vi "Try2.vi"() -> ()   [LabVIEW 2021]
uses:
  Explore/ROS_Subs/ROSCtrl.ctl
panel:
  out "Cmd Line":string
  out "left over fixed":string
  out "Console":string
  in  "Next":bool
  in  "Book":enum32{"Welcome", "lightshow"}(tab)
  in  "Python version":string="3.7"
  in  "Raspberry Pi":T1={"IP Address"="192.168.86.144", "Username"="ubuntu", "password"="iRobot"}
  in  "Update":bool
  in  "LED Colors":u32[](array[colorbox])=[16711680, 327424, 393471, 15699456, 14811391, 64255]
  out "lightshow":string
  # "Welcome to ROS2 for Create3\n\nto get started, enter your IP, hit run,\nand click on Next"
  # "Pick your colors and hit update"
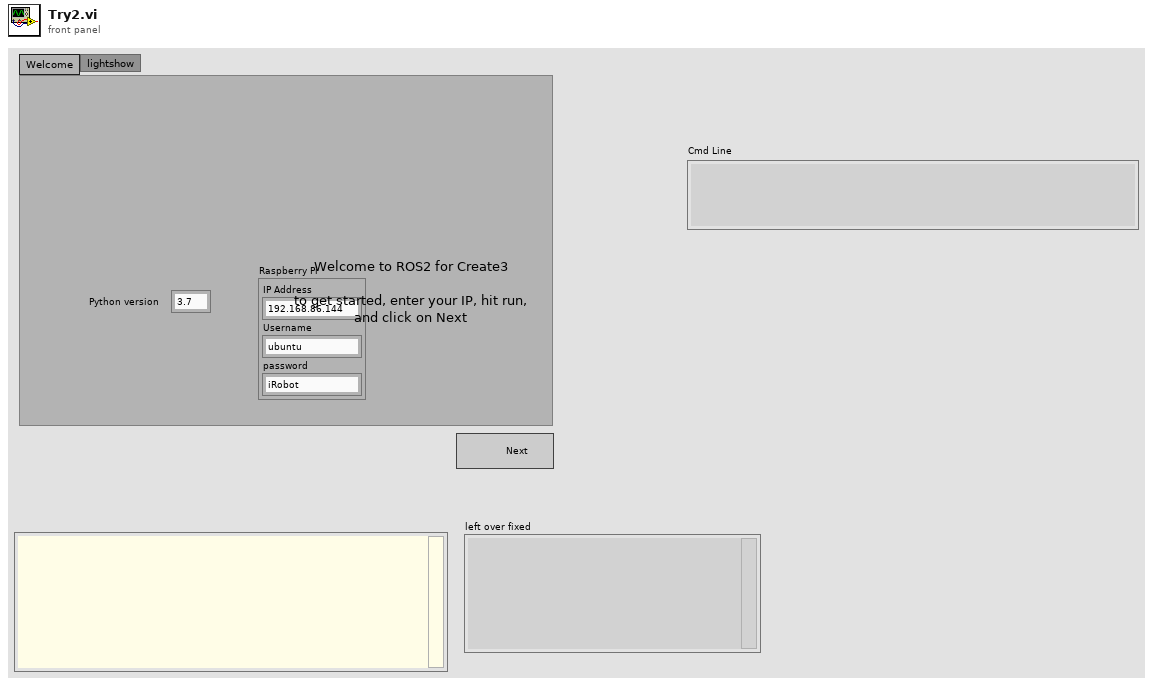
[diagram p1: front panel]
types:
  T1 = cluster{"IP Address":string, "Username":string, "password":string}
  T2 = typedef "ROSCtrl.ctl" = cluster{"Node Name":string, "Topic Name":string, "Message Type":string, "Message":string, "Pub_Time":string}
  T3 = cluster{"override_system":bool, "leds":cluster{"red":u8, "green":u8, "blue":u8}[]}
  T4 = typedef "PythonCtrl.ctl" = cluster{"session":refnum<k35>, "PyPath":path, "Processor":T5, "Port":string, "version":string}
  T5 = typedef "Processors.ctl" = enum16{"SPIKE", "Pi", "Pi_ssh", "OpenMV", "Dunio"}
  T6 = enum8{"Enabled", "Disabled", "Disabled and Grayed Out"}
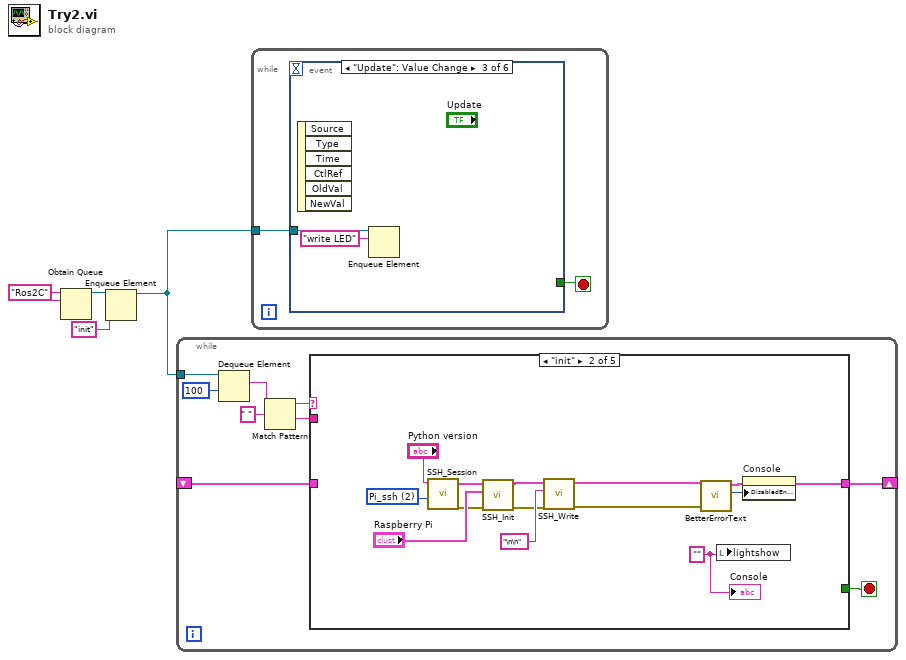
[diagram p0: block diagram]
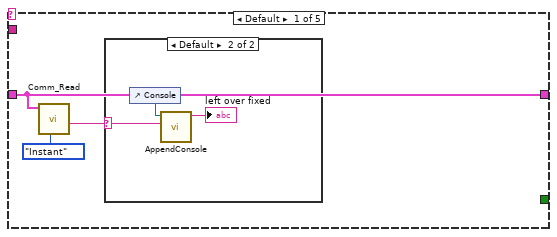
[diagram p2: hidden frame]
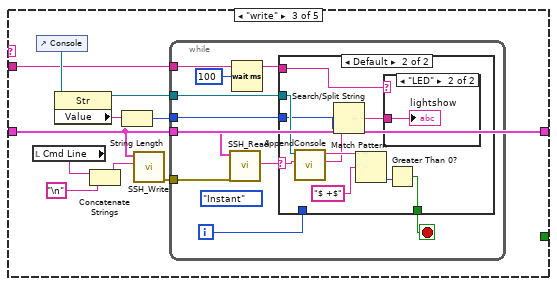
[diagram p4: hidden frame]
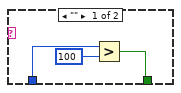
[diagram p5: hidden frame]
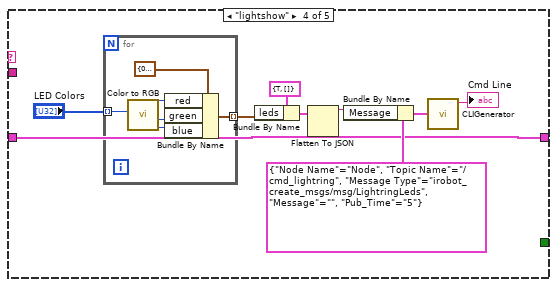
[diagram p7: hidden frame]
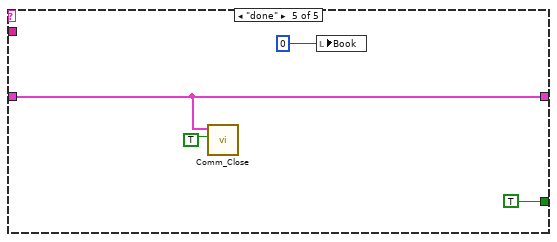
[diagram p8: hidden frame]
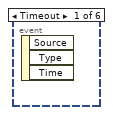
[diagram p9: hidden frame]
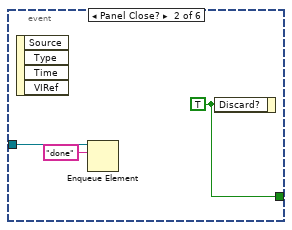
[diagram p10: hidden frame]
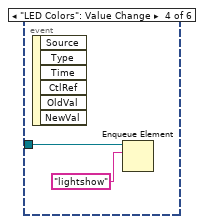
[diagram p11: hidden frame]
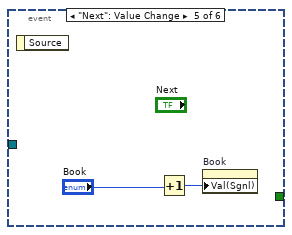
[diagram p12: hidden frame]
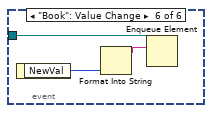
[diagram p13: hidden frame]
diagram:
  w4 = "Ros2C" ("name (unnamed)")
  n1 = Obtain Queue(name (unnamed)=w4, element data type=w4) -> (queue out=w3:refnum<queue>)  [unwired: 3 in, 2 out]
  n2 = Enqueue Element(queue=w3, element="init") -> (queue out=w2:refnum<queue>)  [unwired: 2 in, 2 out]
  n3 = while {
    tunnel: w2 -> [w12]
    shift-right: [w11] -> _
    shift-left: _ -> [w10]
    stop <- w13 stop-if-true
    n4 = Dequeue Element(queue=w12, timeout in ms (-1)=100) -> (element=w8:string)  [unwired: 1 in, 3 out]
    n5 = Match Pattern(string=w8, regular expression=" ") -> (before substring=w6:string, after substring=w5:string)  [unwired: 1 in, 2 out]
    n6 = case shown="\"init\"" w6 {
      tunnel: [_ _ _ _ TRUE ("Discard?")] -> w13
      tunnel: [w15 w31 w35 w65 w81] -> w11
      tunnel: w10 -> [w15 _ w35 w65 w81]
      tunnel: w5 -> [_ _ w36 _ _]
      frame Default {
        n7 = call "Comm_Read.vi"("Task"=enum16{"Instant", "All"}."Instant", "Python"=w15) -> ("Text read"=w14:string)  [unwired: 8 in, 1 out]
        n8 = case shown="Default" w14 {
          selector: w14 -> [_ w19]
          frame "" {
          }
          frame Default {
            n9 = control-ref of="Console"() -> (w18:refnum<vi>)
            n10 = call "AppendConsole.vi"("String"=w19, "String in"=w18) -> ("left over fixed"=→"left over fixed":string)  [unwired: 7 in, 2 out]
          }
        }
      }
      frame "init" {
        w20 = "" ("function name")
        w29 = u16 2 items=["SPIKE", "Pi", "Pi_ssh", "OpenMV", "duino"] ("Processor")
        n11 = call "SSH_Session.vi"("Processor"=w29, "Python version"="Python version") -> ("error out"=w26:errorcluster, "Python"=w28:T4)  [unwired: 8 in]
        n12 = call "SSH_Init.vi"("error in (no error)"=w26, "Raspberry Pi"="Raspberry Pi", "Python in"=w28) -> ("error out"=w23:errorcluster, "Python out"=w25:T4)  [unwired: 6 in, 1 out]
        n13 = call "SSH_Write.vi"("error in (no error)"=w23, "Text to write"="\n\n" ("function name"), "Python"=w25) -> ("error out"=w21:errorcluster, "Python"=w22:T4)  [unwired: 7 in]
        n14 = call "BetterErrorText.vi"("error in (no error)"=w21, "Python"=w22) -> ("Disabled"=w32:T6, "Python out"=w31:T4)  [unwired: 8 in]
        n15 = local write "lightshow"(w20) -> ()
        n16 = property on="Console" class="Str"("DisabledEnum"=w32) -> ()  [unwired: 2 in, 2 out]
        "Console" <- w20
      }
      frame "write" {
        n17 = local read "Cmd Line"() -> (w41:string)
        n18 = control-ref of="Console"() -> (w39:refnum<vi>)
        n19 = property class="Str"(reference=w39) -> ("Value"=w38:string)  [unwired: 1 in, 2 out]
        n20 = Concatenate Strings(w41, "\n" ("function name")) -> (w34:string)
        n21 = String Length(string=w38) -> (length=w37:i32)
        n22 = call "SSH_Write.vi"("Text to write"=w34, "Python"=w35) -> ("error out"=w33:errorcluster)  [unwired: 8 in, 1 out]
        n23 = while {
          tunnel: w35 -> [w44]
          tunnel: w39 -> [w49]
          tunnel: w37 -> [w48]
          tunnel: w36 -> [w45]
          tunnel: w33 -> [w42]
          i -> [w46]
          stop <- w50 stop-if-true
          (unwired) enum16{"Instant", "All"}."Instant" ("Task")
          n24 = call "SSH_Read.vi"("error in (no error)"=w42, "Python"=w44) -> ("Reply"=w43:string)  [unwired: 7 in, 2 out]
          n25 = Wait (ms)(milliseconds to wait=u32 100) -> ()  [unwired: 1 out]
          n26 = case shown="Default" w43 {
            selector: w43 -> [_ w63]
            tunnel: [w51 w60] -> w50
            tunnel: w49 -> [_ w59]
            tunnel: w48 -> [_ w58]
            tunnel: w46 -> [w53 _]
            tunnel: w45 -> [_ w54]
            frame "" {
              n27 = Greater?(x=w53, y=100) -> (0:w51:bool)
            }
            frame Default {
              n28 = call "AppendConsole.vi"("String"=w63, "String in"=w59) -> ("everything"=w55:string, "left over fixed"=w56:string)  [unwired: 7 in, 1 out]
              n29 = Search/Split String(string=w55, offset (0)=w58) -> (match + rest of string=w57:string)  [unwired: 1 in, 2 out]
              n30 = Match Pattern(string=w56, regular expression="$ +$") -> (offset past match=w61:i32)  [unwired: 1 in, 3 out]
              n31 = case shown="\"LED\"" w54 {
                tunnel: w57 -> [_ w64]
                frame Default {
                }
                frame "LED" {
                  "lightshow" <- w64
                }
              }
              n32 = Greater Than 0?(x=w61) -> (x > 0?=w60:bool)
            }
          }
        }
      }
      frame "lightshow" {
        n33 = for {
          tunnel: "LED Colors" -> [w79] mode=indexing
          tunnel: [w74] -> w71 mode=indexing
          n34 = call <vilib>:"Color to RGB.vi"("Color"=w79) -> ("R"=w77:u8, "G"=w76:u8, "B"=w75:u8)  [unwired: 1 out]
          n35 = Bundle By Name(cluster=cluster{"red":u8, "green":u8, "blue":u8} {"red"=0, "green"=0, "blue"=0}, "red"=w77, "green"=w76, "blue"=w75) -> (w74:cluster{"red":u8, "green":u8, "blue":u8})
        }
        n36 = Bundle By Name(cluster=T3 {"override_system"=TRUE, "leds"=[]}, "leds"=w71) -> (w70:T3)
        n37 = Flatten To JSON(anything=w70) -> (JSON string=w69:string)  [unwired: 2 in, 1 out]
        n38 = Bundle By Name(cluster=T2 {"Node Name"="Node", "Topic Name"="/cmd_lightring", "Message Type"="irobot_create_msgs/msg/LightringLeds", "Message"="", "Pub_Time"="5"} ("LED Info"), "Message"=w69) -> (w68:T2)
        n39 = call "CLIGenerator.vi"("ROS Info"=w68) -> ("CLI"=→"Cmd Line":string)  [unwired: 10 in]
      }
      frame "done" {
        n40 = call "Comm_Close.vi"("Show Err?"=TRUE, "Python in"=w81) -> ()  [unwired: 8 in, 2 out]
        n41 = local write "Book"(0) -> ()
      }
    }
  }
  n42 = while {
    tunnel: w2 -> [w84]
    stop <- w85 stop-if-true
    n43 = event shown="[2] \"Update\": Value Change" {
      selector: _ -> [_ _ _ _ _ _]
      dyn-events: _ -> [_ _ _ _ _ _]
      timeout: _ -> [_ _ _ _ _ _]
      tunnel: [_ w88 _ _ _ _] -> w85
      tunnel: w84 -> [_ w87 w90 w92 _ w96]
      event Timeout {
        n44 = event-data() -> ()  [unwired: 1 in, 3 out]
      }
      event Panel Close? {
        w88 = TRUE ("Discard?")
        n45 = event-data() -> ()  [unwired: 1 in, 4 out]
        n46 = Enqueue Element(queue=w87, element="done") -> ()  [unwired: 2 in, 3 out]
        n47 = event-data("Discard?"=w88) -> ()  [unwired: 1 in, 1 out]
      }
      event "Update": Value Change {
        n48 = event-data() -> ()  [unwired: 1 in, 6 out]
        n49 = Enqueue Element(queue=w90, element="write LED") -> ()  [unwired: 2 in, 3 out]
      }
      event "LED Colors": Value Change {
        n50 = event-data() -> ()  [unwired: 1 in, 6 out]
        n51 = Enqueue Element(queue=w92, element="lightshow") -> ()  [unwired: 2 in, 3 out]
      }
      event "Next": Value Change {
        n52 = event-data() -> ()  [unwired: 1 in, 1 out]
        n53 = Increment(x="Book") -> (x+1=w93:enum32{"Welcome", "lightshow"})
        n54 = property on="Book" class="TabCtl (strict)"("Val(Sgnl)"=w93) -> ()  [unwired: 2 in, 2 out]
      }
      event "Book": Value Change {
        n55 = event-data() -> ("NewVal"=w95:enum32{"Welcome", "lightshow"})  [unwired: 1 in]
        n56 = Format Into String(w95) -> (resulting string=w97:string)  [unwired: 3 in, 1 out]
        n57 = Enqueue Element(queue=w96, element=w97) -> ()  [unwired: 2 in, 3 out]
      }
    }
  }
